vi "Create.vi"   [LabVIEW 2021, in "Field_RnD_Services_LIBSSH2_Toolkit.lvlib" / "Agent Identity.lvclass"]
doc: "Creates a new Agent Identity object that represents a libssh2lv shared library Agent Identity struct. This VI must be called, or executed, before using any other Agent Identity-related VIs. This VI allocates memory within the libssh2lv shared library that must be explicitly deallocated, or freed, at the end of the application using the <B>Destroy</B> VI to avoid memory leaks or running Out-of-Memory (OOM) on a resource contrained system.\n\nAn Agent Identity is a SSH username, public/private key, and passphrase/password for a remote SSH/SFTP server stored in a SSH-agent application."
uses:
  220524-VNA RP FLAT.llb/Agent Identity.lvclass
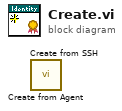
[diagram p0: block diagram]
diagram:
  n1 = call "Create from Agent.vi"() -> ()  [unwired: 9 in, 3 out]
  n2 = call "Create from SSH.vi"() -> ()  [unwired: 10 in, 2 out]
